vi "Page_Source_Configure_TopVI.vi"(8 "error in (no error)":errorcluster, 11 "AB_Source_Exported_Assembly_VI in":refnum<class "AB_Source_Exported_Assembly_VI.lvclass">) -> (0 "error out":errorcluster, 2 "cancelled":bool, 3 "AB_Source_Exported_Assembly_VI out":refnum<class "AB_Source_Exported_Assembly_VI.lvclass">)   [LabVIEW 2020, in "AB_Source_Exported_Assembly_VI.lvclass"]
uses:
  <vilib>/AppBuilder/AB_Classes/Source/ExportedAssemblyVI/AB_Source_Exported_Assembly_VI.lvclass
  e:/builds/penguin/labview/branches/2020/dev/dist/vi.lib/AppBuilder/AB_Classes/Source/AB_Source.lvclass
  <vilib>/AppBuilder/AB_Classes/Build/AB_Build.lvclass
  <vilib>/AppBuilder/AB_Classes/Source/AB_Source.lvclass
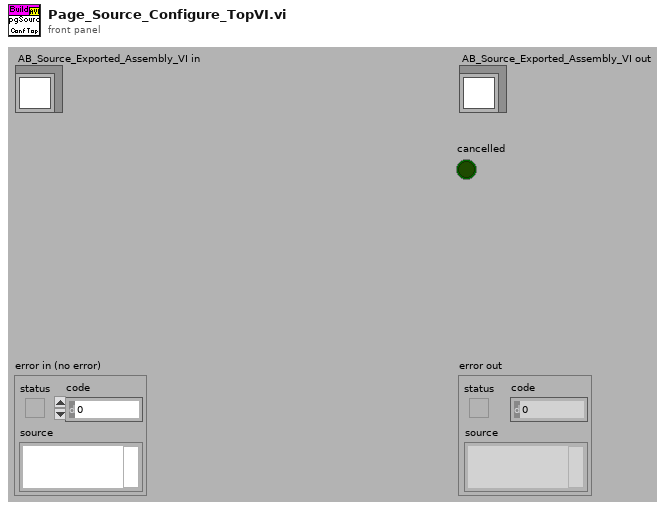
[diagram p1: front panel]
types:
  T1 = typedef "AB_InteropAssembly_DistVI_Proto_Info.ctl" = cluster{"Library Name":string, "VI Name":string, "Method Name":string, "LV Class":path, "Param Names":string[], "Data Types":string[], "Dirs":T2[], "InputIdx":i32[], "OutputIdx":i32[], "ConNum":i8[], "IsCustomDocumentation":bool, "Custom Documentation":string, "IsProtected":bool, "IsSanitized":bool}
  T2 = typedef "IOStatus.ctl" = enum16{"Input", "Output", "Input/Output", "InputDeleted", "OutputDeleted", "IODeleted", "ErrorClusterIn", "ErrorClusterOut"}
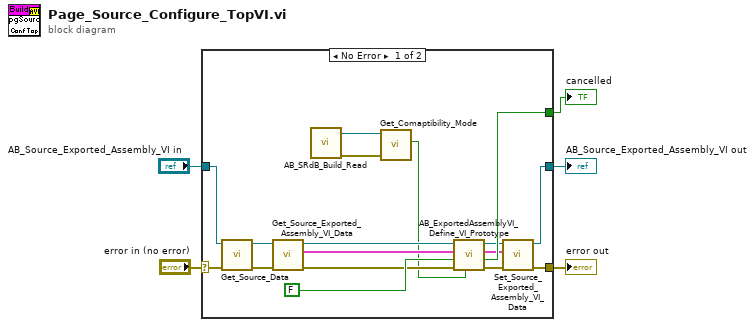
[diagram p0: block diagram]
diagram:
  n1 = case shown="No Error" "error in (no error)" {
    selector: "error in (no error)" -> [w21 w24]
    tunnel: "AB_Source_Exported_Assembly_VI in" -> [w22 w23]
    tunnel: [w17 w23] -> w4
    tunnel: [w15 w24] -> w2
    tunnel: [w19 _] -> w1
    frame No Error {
      n2 = call <vilib>:"Get_Source_Data.vi"("error in (no error)"=w21, "Class in"=w22) -> ("error out"=w12:errorcluster, "Class out"=w14:refnum<class "AB_Source_Exported_Assembly_VI.lvclass">)  [unwired: 8 out]
      n3 = call <vilib>:"Get_Source_Exported_Assembly_VI_Data.vi"("error in (no error)"=w12, "AB_Source_Exported_Assembly_VI.lvclass in"=w14) -> ("error out"=w11:errorcluster, "ExportAssemblyVIinfo"=w13:T1, "AB_Source_Exported_Assembly_VI.lvclass out"=w10:refnum<class "AB_Source_Exported_Assembly_VI.lvclass">)  [unwired: 7 out]
      n4 = call <resource>:"AB_SRdB_Build_Read.vi"() -> ("error out"=w8:errorcluster, "build out"=w6:refnum<class "AB_Build.lvclass">)  [unwired: 1 in, 9 out]
      n5 = call-dynamic "Get_Comaptibility_Mode.vi"("error in (no error)"=w8, "AB_Build in"=w6) -> ("CompatibilityWith2011"=w7:bool)  [unwired: 7 in, 2 out]
      n6 = call <vilib>:"AB_ExportedAssemblyVI_Define_VI_Prototype.vi"("LV2011Compatibility"=w7, "error in"=w11, "verify only"=FALSE, "ExportAssemblyVIinfo in"=w13, "AB_Source_Exported_Assembly_VI.lvclass"=w10) -> ("error out"=w16:errorcluster, "Cancel"=w19:bool, "ExportAssemblyVIinfo out"=w18:T1, "AB_Source_Exported_Assembly_VI.lvclass Out"=w9:refnum<class "AB_Source_Exported_Assembly_VI.lvclass">)  [unwired: 3 out]
      n7 = call <vilib>:"Set_Source_Exported_Assembly_VI_Data.vi"("error in (no error)"=w16, "ExportAssemblyVIinfo"=w18, "AB_Source_Exported_Assembly_VI.lvclass in"=w9) -> ("error out"=w15:errorcluster, "AB_Source_Exported_Assembly_VI.lvclass out"=w17:refnum<class "AB_Source_Exported_Assembly_VI.lvclass">)  [unwired: 7 out]
    }
    frame Error {
    }
  }
  "error out" <- w2
  "AB_Source_Exported_Assembly_VI out" <- w4
  "cancelled" <- w1
